vi "离线每组字节.vi"(8 "错误输入":errorcluster caption="输出簇", 11 "文件句柄":i32) -> (0 "错误输出":errorcluster, 2 "每组字节数":i32, 3 "文件句柄出":i32)   [LabVIEW 2011]
uses:
  dll/em9636.dll
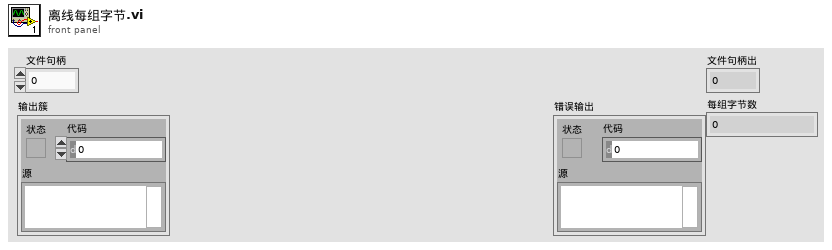
[diagram p1: front panel]
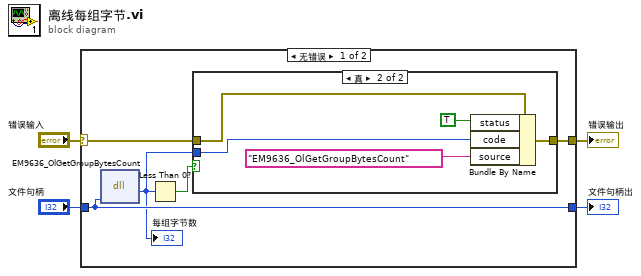
[diagram p0: block diagram]
diagram:
  n1 = case shown="无错误" "错误输入" {
    selector: "错误输入" -> [w6 w17]
    tunnel: [w8 w17] -> w3
    tunnel: "文件句柄" -> [w7 w16]
    tunnel: [w7 w16] -> w1
    frame No Error {
      n2 = dll-call lib="PTH1abs Eèµ éç LABVIEWæºVI(v2.0)EM9636BD)EM9636BDè°ç¨APIå½æ°æ¹æ³éè®¯ä¾ç¨EM9636labview8.5-1511048.5dll\nem9636.dll" fn="EM9636_OlGetGroupBytesCount"("文件句柄"=w7) -> ("每组字节"=w5:i32)  [unwired: 4 in, 2 out]
      "每组字节数" <- w5
      n3 = Less Than 0?(x=w5) -> (x < 0?=w9:bool)
      n4 = case shown="真" w9 {
        tunnel: [w10 w13] -> w8
        tunnel: w6 -> [w10 w15]
        tunnel: w5 -> [_ w12]
        frame False {
        }
        frame True {
          n5 = Bundle By Name(cluster=w15, "status"=TRUE, "code"=w12, "source"="EM9636_OlGetGroupBytesCount") -> (w13:errorcluster)
        }
      }
    }
    frame Error {
    }
  }
  "文件句柄出" <- w1
  "错误输出" <- w3
